vi "Delete Row.vi"(11 "board array in":u8[][](array[numeric])) -> (0 "Rows Deleted":u16, 3 "board array out":u8[][](array[numeric]))   [LabVIEW 2019]
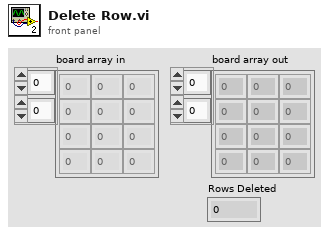
[diagram p1: front panel]
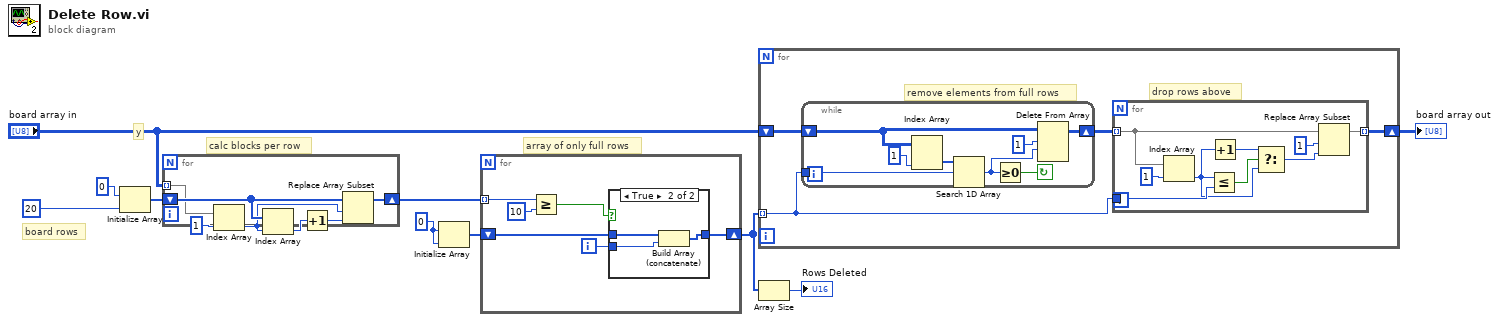
[diagram p0: block diagram]
diagram:
  w5 = 0
  # "array of only full rows"
  # "calc blocks per row"
  # "y"
  # "board rows"
  n1 = Initialize Array(0, 20) -> (w8:i32[])
  n2 = for {
    tunnel: "board array in" -> [w13] mode=indexing
    shift-right: [w14] -> w7
    shift-left: w8 -> [w16]
    n3 = Index Array(array=w13, index=1) -> (element=w11:u8)
    n4 = Index Array(array=w16, index=w11) -> (element=w17:i32)
    n5 = Increment(x=w17) -> (x+1=w15:i32)
    n6 = Replace Array Subset(array=w16, new element=w15, index=w11) -> (w14:i32[])
  }
  n7 = Initialize Array(w5, w5) -> (w6:i32[])
  n8 = for {
    tunnel: w7 -> [w22] mode=indexing
    shift-right: [w18] -> w2
    shift-left: w6 -> [w20]
    i -> [w19]
    n9 = Greater Or Equal?(x=w22, y=10) -> (x >= y?=w21:bool)
    n10 = case shown="True" w21 {
      tunnel: w20 -> [w24 w27]
      tunnel: w19 -> [_ w26]
      tunnel: [w24 w25] -> w18
      frame False {
      }
      frame True {
        n11 = Build Array (concatenate)(w27, w26) -> (w25:i32[])
      }
    }
  }
  n12 = for {
    shift-right: [w29] -> w3
    shift-left: "board array in" -> [w31]
    tunnel: w2 -> [w28] mode=indexing
    # "drop rows above"
    # "remove elements from full rows"
    n13 = while {
      shift-right: [w43] -> w30
      shift-left: w31 -> [w45]
      tunnel: w28 -> [w41]
      stop <- w46 continue-if-true
      n14 = Index Array(array=w45, index (col)=1) -> (element=w47:u8[])  [unwired: 1 in]
      n15 = Search 1D Array(1D array=w47, element=w41) -> (index of element=w42:i32)  [unwired: 1 in]
      n16 = Greater Or Equal To 0?(x=w42) -> (x >= 0?=w46:bool)
      n17 = Delete From Array(array=w45, length=1, index (row)=w42) -> (array with subset deleted=w43:u8[][])  [unwired: 1 in, 1 out]
    }
    n18 = for {
      tunnel: w30 -> [w33] mode=indexing
      tunnel: w28 -> [w39]
      tunnel: [w32] -> w29 mode=indexing
      n19 = Index Array(array=w33, index=1) -> (element=w36:u8)
      n20 = Less Or Equal?(x=w36, y=w39) -> (x <= y?=w38:bool)
      n21 = Increment(x=w36) -> (x+1=w37:u8)
      n22 = Select(t=w37, s=w38, f=w36) -> (s? t:f=w35:u8)
      n23 = Replace Array Subset(array=w33, new element=w35, index=1) -> (w32:u8[])
    }
  }
  "board array out" <- w3
  n24 = Array Size(array=w2) -> (size(s)=→"Rows Deleted":i32)
